vi "Format SmartCOM Message.vi"(0 "Message":string, 1 "Param 1":string, 2 "Param 2":string, 3 "Params":string[](array[string]), 4 "Name":string) -> (14 "Message to Send":string)   [LabVIEW 2017]
uses:
  <vilib>/regexp/Match Regular Expression.xnode
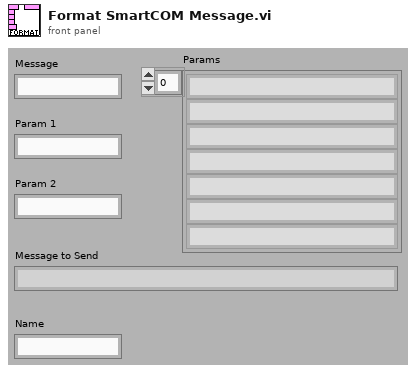
[diagram p1: front panel]
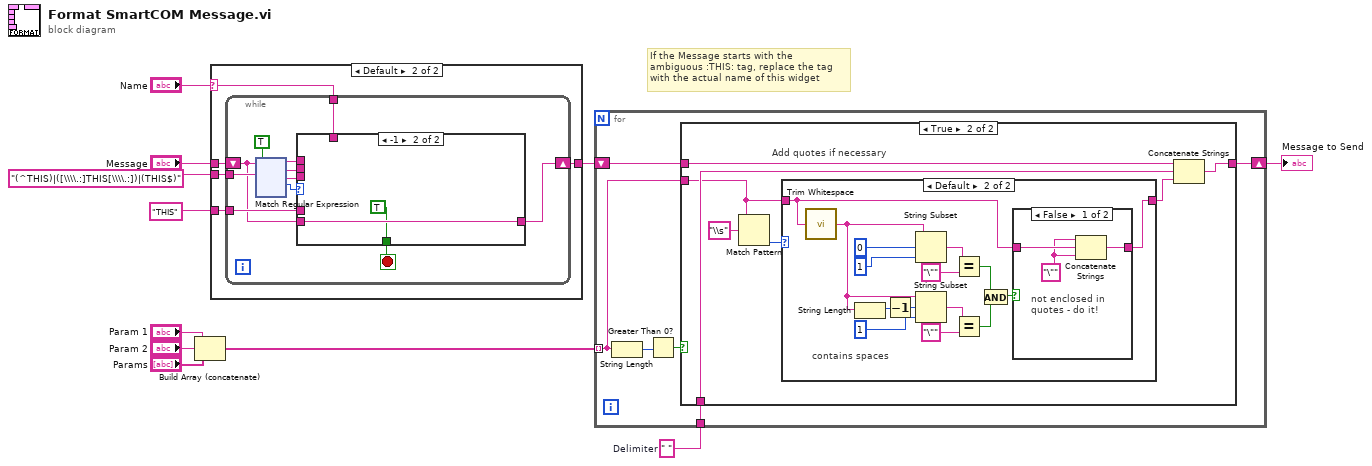
[diagram p0: block diagram]
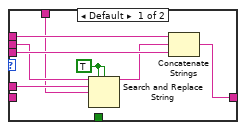
[diagram p3: hidden frame]
diagram:
  w11 = " "  # Delimiter
  # "If the Message starts with the ambiguous :THIS: tag, replace the tag with the actual name of this widget"
  n1 = Build Array (concatenate)("Param 1", "Param 2", "Params") -> (w5:string[])
  n2 = case shown="Default" "Name" {
    selector: "Name" -> [_ w13]
    tunnel: [w12 w17] -> w10
    tunnel: "Message" -> [w12 w16]
    tunnel: "(^THIS)|([\\\\.:]THIS[\\\\.:])|(THIS$)" ("regex") -> [_ w15]
    tunnel: "THIS" ("regex") -> [_ w14]
    frame "" {
    }
    frame Default {
      n3 = while {
        tunnel: w15 -> [w27]
        shift-right: [w19] -> w17
        shift-left: w16 -> [w18]
        tunnel: w14 -> [w21]
        tunnel: w13 -> [w20]
        stop <- w26 stop-if-true
        n4 = xnode "Match Regular Expression"("input string"=w18, "regular expression"=w27, "ignore case? (F)"=TRUE ("replace all? (F)")) -> ("before match"=w25:string, "whole match"=w24:string, "after match"=w23:string, "offset past match"=w22:i32)  [unwired: 2 in, 2 out]
        n5 = case shown="-1" w22 {
          tunnel: [w34 w38] -> w19
          tunnel: w18 -> [_ w38]
          tunnel: w25 -> [w36 _]
          tunnel: w24 -> [w33 _]
          tunnel: w23 -> [w35 _]
          tunnel: [_ TRUE] -> w26
          tunnel: w21 -> [w31 _]
          tunnel: w20 -> [w30 _]
          frame Default {
            w29 = TRUE ("replace all? (F)")
            n6 = Search and Replace String(replace all?=w29, case sensitive?=w29, input string=w33, search string=w31, replace string=w30) -> (result string=w32:string)  [unwired: 1 in, 5 out]
            n7 = Concatenate Strings(w36, w32, w35) -> (w34:string)
          }
          frame -1 {
          }
        }
      }
    }
  }
  n8 = for {
    shift-right: [w152] -> w2
    shift-left: w10 -> [w153]
    tunnel: w5 -> [w151] mode=indexing
    tunnel: w11 -> [w150]
    n9 = String Length(string=w151) -> (length=w155:i32)
    n10 = Greater Than 0?(x=w155) -> (x > 0?=w154:bool)
    n11 = case shown="True" w154 {
      tunnel: [w156 w162] -> w152
      tunnel: w153 -> [w156 w163]
      tunnel: w151 -> [_ w158]
      tunnel: w150 -> [_ w161]
      frame False {
      }
      frame True {
        # "Add quotes if necessary"
        n12 = Match Pattern(string=w158, regular expression="\\s") -> (offset past match=w159:i32)  [unwired: 4 out]
        n13 = case shown="Default" w159 {
          tunnel: w158 -> [w164 w166]
          tunnel: [w164 w165] -> w157
          frame -1 {
            # "no spaces"
          }
          frame Default {
            # "contains spaces"
            n14 = call <vilib>:"Trim Whitespace.vi"("string"=w166) -> ("trimmed string"=w168:string)  [unwired: 1 in]
            n15 = String Length(string=w168) -> (length=w172:i32)
            n16 = Decrement(x=w172) -> (x-1=w171:i32)
            n17 = String Subset(string=w168, offset (0)=0, length (rest)=1 ("length (rest)")) -> (substring=w175:string)
            n18 = String Subset(string=w168, offset (0)=w171, length (rest)=1 ("length (rest)")) -> (substring=w176:string)
            n19 = Equal?(x=w175, y="\"") -> (x = y?=w170:bool)
            n20 = Equal?(x=w176, y="\"") -> (x = y?=w169:bool)
            n21 = And(x=w170, y=w169) -> (x .and. y?=w167:bool)
            n22 = case shown="False" w167 {
              tunnel: w166 -> [w181 w183]
              tunnel: [w182 w183] -> w165
              frame False {
                w180 = "\"" ("y")
                # "not enclosed in\nquotes - do it!"
                n23 = Concatenate Strings(w180, w181, w180) -> (w182:string)
              }
              frame True {
                # "already enclosed\nin quotes"
              }
            }
          }
        }
        n24 = Concatenate Strings(w163, w161, w157) -> (w162:string)
      }
    }
  }
  "Message to Send" <- w2
